vi "HFRR ADV v11.vi"() -> ()   [LabVIEW 2025] (continued)
            n1532 = local read "AIR TEMP INTERCEPT:"() -> (w2037:dbl)
            n1533 = case shown="\"0\", Default" "Calibrating" {
              tunnel: w2028 -> [w2082 _]
              tunnel: [w2082 w2083] -> w2027
              tunnel: w2026 -> [_ w2083]
              frame "0", Default {
              }
              frame "1" {
              }
            }
            n1534 = Multiply(x=w2016, y="ECR_Gain") -> (x*y=w2015:dbl)
            n1535 = Add(x=w2022, y=w2033) -> (x+y=w2038:dbl)
            n1536 = Multiply(x=w2056, y=79.77669138) -> (x*y=w2054:dbl)
            n1537 = Select(t=0.01 ("FF fil1"), s=w2053, f=0.1 ("FF fil1")) -> (s? t:f=w2049:dbl)
            n1538 = local read "ecr"() -> (w2010:dbl)
            n1539 = Multiply(x=w2021, y=w2041) -> (x*y=w2023:dbl)
            n1540 = Multiply(x=w2063, y=w2054) -> (x*y=w2060:dbl[])
            n1541 = Multiply(x=w2015, y=0.2) -> (x*y=w2008:dbl)
            n1542 = Multiply(x=0.8, y=w2010) -> (x*y=w2009:dbl)
            n1543 = call <vilib>:"Mean PtByPt.vi"("x"=w2038, "sample length"=10) -> ("mean"=w1999:dbl)  [unwired: 2 in, 1 out]
            "TEMP 2" <- w1999
            "TEMP 3" <- w1999
            n1544 = local read "AIR TEMP"() -> (w2046:dbl)
            n1545 = Add(x=w2023, y=w2037) -> (x+y=w2039:dbl)
            n1546 = call-poly <vilib>:"Mean.vi"("X"=w2060) -> ("mean"=w2061:dbl)  [unwired: 1 out]
            n1547 = Add(x=w2008, y=w2009) -> (x+y=w2007:dbl)
            n1548 = Subtract(x=1.0 ("y"), y=w2049) -> (x-y=w2047:dbl)
            n1549 = local write "TEMP"(w1999) -> ()
            n1550 = Multiply(x=w2047, y=w2046) -> (x*y=w2045:dbl)
            n1551 = Multiply(x=w2039, y=w2049) -> (x*y=w2050:dbl)
            n1552 = Not A Number/Path/Refnum?(number/path/refnum=w2007) -> (NaN/Path/Refnum?=w2017:bool)
            n1553 = Subtract(x=w2060, y=w2061) -> (x-y=w2032:dbl[])
            n1554 = local read "FRICVALZ"() -> (w2070:dbl)
            n1555 = case shown="True" "Camera Button" {
              tunnel: w2027 -> [_ w2089]
              tunnel: "Standard Temp. ( °c )" -> [_ w2088]
              frame False {
              }
              frame True {
                n1556 = Build Array(w2088, w2089) -> (w2087:dbl[])
                n1557 = local write "Camera Button"(FALSE ("Boolean 4")) -> ()
                n1558 = local read "Captured Values"() -> (w2086:dbl[][])
                n1559 = Build Array (concatenate)(w2086, w2087) -> (w2084:dbl[][])
                n1560 = local write "Captured Values"(w2084) -> ()
              }
            }
            n1561 = Compound Arithmetic op=OR("FRICVALZ 4", "FRICVALZ 3", "FRICVALZ 2") -> (w2001:bool)
            n1562 = Add(x=w2050, y=w2045) -> (x+y=w2043:dbl)
            n1563 = Absolute Value(x=w2032) -> (abs(x)=w2065:dbl[])
            n1564 = call-poly <vilib>:"RMS.vi"("X"=w2032) -> ("rms value"=w2031:dbl)  [unwired: 1 out]
            n1565 = Select(t=0.0, s=w2017, f=w2007) -> (s? t:f=w2014:dbl)
            n1566 = call-poly <vilib>:"Mean.vi"("X"=w2065) -> ()  [unwired: 2 out]
            n1567 = local read "FF 2"() -> (w2072:dbl)
            n1568 = case shown="True" w2001 {
              tunnel: w2031 -> [_ w2094]
              frame False {
              }
              frame True {
                w2093 = FALSE ("FRICVALZ")
                n1569 = local write "FRICVALZ 3"(w2093) -> ()
                n1570 = local write "FRICVALZ 2"(w2093) -> ()
                n1571 = local write "FRICVALZ 4"(w2093) -> ()
                "FRICVALZ" <- w2094
              }
            }
            n1572 = Subtract(x=w2031, y=w2070) -> (x-y=w2064:dbl)
            n1573 = Not A Number/Path/Refnum?(number/path/refnum=w2043) -> (NaN/Path/Refnum?=w2044:bool)
            n1574 = In Range and Coerce(upper limit=100.0, x=w2014, lower limit=0.0) -> ()  [unwired: 2 out]
            n1575 = Select(t=0.0, s=w2044, f=w2043) -> (s? t:f=w2004:dbl)
            "AIR TEMP" <- w2004
            n1576 = Multiply(x=w2064, y=0.1 ("FF fil1")) -> (x*y=w2076:dbl)
            n1577 = Multiply(x=0.9 ("FF fil2"), y=w2072) -> (x*y=w2075:dbl)
            n1578 = disable-structure shown="Disabled" {
              frame Disabled {
                n1579 = local read "NORMAL LOAD"() -> ()  [unwired: 1 out]
              }
              frame Enabled {
              }
            }
            n1580 = call "Elapsed Time11"("Time Target (s)"=1.0) -> ("Time has Elapsed"=w2006:bool)  [unwired: 11 in, 7 out]
            n1581 = Add(x=w2076, y=w2075) -> (x+y=w1994:dbl)
            "FF 2" <- w1994
            "FF 4" <- w1994
            n1582 = case shown="True" w2006 {
              tunnel: w2004 -> [_ w2078]
              frame False {
              }
              frame True {
                "AirT" <- w2078
              }
            }
            n1583 = local read "TEMP"() -> (w2069:dbl)
            n1584 = local write "FF 3"(w1994) -> ()
            n1585 = Not A Number/Path/Refnum?(number/path/refnum=w1994) -> (NaN/Path/Refnum?=w2067:bool)
            n1586 = Divide(x=w1994, y=1.96) -> (x/y=w2034:dbl)
            n1587 = Not A Number/Path/Refnum?(number/path/refnum=w2069) -> (NaN/Path/Refnum?=w2068:bool)
            n1588 = Compound Arithmetic op=OR(w2068, w2067) -> (w2066:bool)
            n1589 = Not A Number/Path/Refnum?(number/path/refnum=w2034) -> (NaN/Path/Refnum?=w2035:bool)
            n1590 = case shown="True" w2066 {
              frame False {
              }
              frame True {
                n1591 = local write "TEMP"(0.0 ("TEMP")) -> ()
                n1592 = local write "FF 2"(0.0 ("FF 2")) -> ()
                n1593 = local write "reinit"(TRUE ("reinit")) -> ()
              }
            }
            n1594 = Select(t=0.0, s=w2035, f=w2034) -> (s? t:f=w1995:dbl)
            "COF 2" <- w1995
            n1595 = local write "COF 3"(w1995) -> ()
          }
          frame #4 {
            n1596 = flat-sequence {
              frame #0 {
                n1597 = Wait (ms)(milliseconds to wait=u32 100) -> ()  [unwired: 1 out]
              }
              frame #1 {
                n1598 = local write "Lift"(FALSE ("Lift")) -> ()
              }
            }
            n1599 = case shown="True" "Calculate Button" {
              frame False {
              }
              frame True {
                n1600 = local write "Calculate Button"(FALSE ("Boolean 6")) -> ()
                n1601 = local read "Captured Values"() -> (w2105:dbl[][])
                n1602 = Index Array(array=w2105, index (col) #1=0 ("disabled index (col)"), index (col) #2=1 ("index (col)")) -> (element #1=w2103:dbl[], element #2=w2101:dbl[])  [unwired: 2 in]
                n1603 = call <vilib>:"Linear Fit.vi"("Y"=w2103, "X"=w2101) -> ("Best Linear Fit"=→"Best Fit":dbl[], "slope"=w2097:dbl, "intercept"=w2096:dbl)  [unwired: 9 in, 2 out]
                "Slope" <- w2097
                "Intercept" <- w2096
                n1604 = local read "Calibrating"() -> (w2098:string)
                n1605 = case shown="\"1\"" w2098 {
                  tunnel: w2097 -> [w2107 w2109]
                  tunnel: w2096 -> [w2106 w2108]
                  frame "0", Default {
                    n1606 = local write "TEMPERATURE :"(w2107) -> ()
                    n1607 = local write "TEMP INTERCEPT:"(w2106) -> ()
                  }
                  frame "1" {
                    n1608 = local write "AIR TEMPERATURE :"(w2109) -> ()
                    n1609 = local write "AIR TEMP INTERCEPT:"(w2108) -> ()
                  }
                }
              }
            }
          }
        }
      }
    }
    n1610 = Wait (ms)(milliseconds to wait=u32 50) -> ()  [unwired: 1 out]
    n1611 = local read "Quit"() -> (w1899:bool)
    "Rate" <- 2500.0 ("No of Samples")
    "Humid Last buf" <- dbl[] [0.0, 0.0, 0.0, 0.0] ("Humid Last buf")
  }
  n1612 = while {
    tunnel: w60 -> [_]
    tunnel: [w2139] -> _
    tunnel: [w2114] -> w57
    i -> [w2139]
    stop <- w2114 stop-if-true
    # "C:\\LAB-IQ-NXT\\Scar View.exe"
    n1613 = local read "OK Button 16"() -> (w2128:bool)
    n1614 = local read "Re-Initialise"() -> (w2124:bool)
    n1615 = local read "Main Tab"() -> (w2120:T2)
    n1616 = local read "service 3"() -> (w2121:bool)
    n1617 = local read "OPEN 6"() -> (w2123:bool)
    n1618 = local read "EDIT 2"() -> (w2126:bool)
    n1619 = flat-sequence {
      frame #0 {
        n1620 = local read "SAVE 2"() -> (w2742:bool)
        n1621 = stacked-sequence {
          frame #0 {
            n1622 = local read "EDIT"() -> (w2796:bool)
            n1623 = case shown="True" w2796 {
              tunnel: [u8 2 ("Disabled") u8 0 ("Disabled")] -> _
              frame False {
                w2798 = FALSE
                n1624 = local write "Password"("") -> ()
                n1625 = property on="SrvM CP" class="Bool (strict)"("Visible"=w2798) -> ()  [unwired: 2 in, 2 out]
                n1626 = property on="message" class="Str"("Visible"=w2798) -> ()  [unwired: 2 in, 2 out]
                n1627 = local write "x = y?"(w2798) -> ()
                n1628 = property on="Password" class="Str"("Visible"=w2798) -> ()  [unwired: 2 in, 2 out]
                n1629 = property on="ENTER THE NEW PASSWORD" class="Str"("Visible"=w2798) -> ()  [unwired: 2 in, 2 out]
                n1630 = property on="ENTER CURRENT PASSWORD" class="Str"("Visible"=w2798) -> ()  [unwired: 2 in, 2 out]
                n1631 = local write "SrvM CP"(w2798) -> ()
              }
              frame True {
                w2801 = TRUE
                n1632 = property on="SrvM CP" class="Bool (strict)"("Visible"=w2801) -> ()  [unwired: 2 in, 2 out]
                n1633 = property on="Password" class="Str"("Visible"=w2801) -> ()  [unwired: 2 in, 2 out]
              }
            }
            "dipl pwd" <- "@143$\n" ("dipl pwd")
          }
          frame #1 {
            # "Gain password"
            n1634 = String To Byte Array(string="ENTER CURRENT PASSWORD") -> (unsigned byte array=w2806:u8[])
            n1635 = Search 1D Array(1D array=w2806, element=u8 10) -> (index of element=w2809:i32)  [unwired: 1 in]
            n1636 = Index Array(array=w2806, index=w2809) -> (element=w2805:u8)
            n1637 = Equal?(x=w2805, y=10) -> (x = y?=w2803:bool)
            n1638 = case shown="True" w2803 {
              frame False {
                n1639 = property on="ENTER THE NEW PASSWORD" class="Str"("Visible"=FALSE) -> ()  [unwired: 2 in, 2 out]
              }
              frame True {
                # "password"
                # "change password logic"
                n1640 = local read "ENTER CURRENT PASSWORD"() -> (w2822:string)
                n1641 = local read "dipl pwd"() -> (w2816:string)
                n1642 = String To Byte Array(string=w2822) -> (unsigned byte array=w2824:u8[])
                n1643 = String To Byte Array(string=w2816) -> (unsigned byte array=w2817:u8[])
                n1644 = Array Size(array=w2824) -> (size(s)=w2821:i32)
                n1645 = Array Size(array=w2817) -> (size(s)=w2819:i32)
                n1646 = for {
                  N: w2821 -> [_]
                  tunnel: w2824 -> [w2848]
                  tunnel: [w2846] -> w2825 mode=indexing
                  tunnel: w2821 -> [w2840]
                  i -> [w2841]
                  n1647 = Decrement(x=w2840) -> (x-1=w2838:i32)
                  n1648 = Equal?(x=w2841, y=w2838) -> (x = y?=w2839:bool)
                  n1649 = Index Array(array=w2848, index=w2841) -> (element=w2842:u8)
                  n1650 = Number To Decimal String(number=w2842) -> (decimal integer string=w2847:string)  [unwired: 1 in]
                  n1651 = Select(t="", s=w2839, f="\r") -> (s? t:f=w2844:string)
                  n1652 = Concatenate Strings(w2847, w2844) -> (w2846:string)
                }
                n1653 = for {
                  N: w2819 -> [_]
                  tunnel: w2817 -> [w2836]
                  tunnel: [w2834] -> w2818 mode=indexing
                  tunnel: w2819 -> [w2831]
                  i -> [w2832]
                  n1654 = Decrement(x=w2831) -> (x-1=w2830:i32)
                  n1655 = Equal?(x=w2832, y=w2830) -> (x = y?=w2829:bool)
                  n1656 = Index Array(array=w2836, index=w2832) -> (element=w2835:u8)
                  n1657 = Number To Decimal String(number=w2835) -> (decimal integer string=w2833:string)  [unwired: 1 in]
                  n1658 = Select(t="", s=w2829, f="\r") -> (s? t:f=w2826:string)
                  n1659 = Concatenate Strings(w2833, w2826) -> (w2834:string)
                }
                n1660 = local read "string"() -> (w2823:string)
                n1661 = Concatenate Strings(w2818) -> (w2812:string)
                n1662 = Concatenate Strings(w2823) -> (w2820:string)
                n1663 = Concatenate Strings(w2825) -> (w2813:string)
                n1664 = Equal?(x=w2813, y=w2820) -> (x = y?=w2815:bool)
                n1665 = Equal?(x=w2813, y=w2812) -> (x = y?=w2811:bool)
                n1666 = Or(x=w2815, y=w2811) -> (x .or. y?=w2814:bool)
                n1667 = case shown="True" w2814 {
                  frame False {
                  }
                  frame True {
                    n1668 = property on="ENTER THE NEW PASSWORD" class="Str"("Visible"=TRUE) -> ()  [unwired: 2 in, 2 out]
                  }
                }
              }
            }
          }
          frame #2 {
            n1669 = String To Byte Array(string="ENTER THE NEW PASSWORD") -> (unsigned byte array=w2851:u8[])
            n1670 = Search 1D Array(1D array=w2851, element=u8 10) -> (index of element=w2855:i32)  [unwired: 1 in]
            n1671 = Index Array(array=w2851, index=w2855) -> (element=w2853:u8)
            n1672 = Equal?(x=w2853, y=10) -> (x = y?=w2850:bool)
            n1673 = case shown="False" w2850 {
              frame False {
              }
              frame True {
                n1674 = local write "EDIT"(FALSE) -> ()
                n1675 = local write "SrvM CP"(FALSE) -> ()
                n1676 = local read "ENTER THE NEW PASSWORD"() -> (w2858:string)
                n1677 = String To Byte Array(string=w2858) -> (unsigned byte array=w2863:u8[])
                n1678 = Array Size(array=w2863) -> (size(s)=w2860:i32)
                n1679 = for {
                  N: w2860 -> [_]
                  tunnel: w2863 -> [w2876]
                  tunnel: [w2873] -> w2865 mode=indexing
                  tunnel: w2860 -> [w2868]
                  i -> [w2866]
                  n1680 = Decrement(x=w2868) -> (x-1=w2869:i32)
                  n1681 = Equal?(x=w2866, y=w2869) -> (x = y?=w2870:bool)
                  n1682 = Index Array(array=w2876, index=w2866) -> (element=w2875:u8)
                  n1683 = Number To Decimal String(number=w2875) -> (decimal integer string=w2874:string)  [unwired: 1 in]
                  n1684 = Select(t="", s=w2870, f="\r") -> (s? t:f=w2867:string)
                  n1685 = Concatenate Strings(w2874, w2867) -> (w2873:string)
                }
                n1686 = local read "file path"() -> (w2857:path)
                n1687 = Concatenate Strings(w2865) -> (w2859:string)
                n1688 = Delete(path (use dialog)=w2857) -> (deleted path=w2861:path)  [unwired: 4 in, 2 out]
                n1689 = call <vilib>:"Write Characters To File.vi"("append to file? (new file:F)"=FALSE, "character string"=w2859, "file path (dialog if empty)"=w2861) -> ()  [unwired: 2 in, 1 out]
              }
            }
          }
          frame #3 {
            n1690 = case shown="True" "SrvM CP" {
              frame False {
                w2879 = ""
                n1691 = local write "ENTER CURRENT PASSWORD"(w2879) -> ()
                n1692 = local write "ENTER THE NEW PASSWORD"(w2879) -> ()
                n1693 = property on="ENTER CURRENT PASSWORD" class="Str"("Visible"=FALSE) -> ()  [unwired: 2 in, 2 out]
              }
              frame True {
                n1694 = property on="ENTER THE NEW PASSWORD" class="Str"() -> ("Visible"=w2880:bool)  [unwired: 2 in, 2 out]
                n1695 = Not(x=w2880) -> (.not. x?=w2881:bool)
                n1696 = property on="ENTER CURRENT PASSWORD" class="Str"("Visible"=w2881) -> ()  [unwired: 2 in, 2 out]
              }
            }
          }
          frame #4 {
            n1697 = String To Byte Array(string="Password") -> (unsigned byte array=w2888:u8[])
            n1698 = Search 1D Array(1D array=w2888, element=u8 10) -> (index of element=w2886:i32)  [unwired: 1 in]
            n1699 = Index Array(array=w2888, index=w2886) -> (element=w2887:u8)
            n1700 = Equal?(x=w2887, y=10) -> (x = y?=w2883:bool)
            n1701 = case shown="True" w2883 {
              frame False {
              }
              frame True {
                # "password"
                # "password"
                n1702 = local read "Password"() -> (w2901:string)
                n1703 = String To Byte Array(string=w2901) -> (unsigned byte array=w2904:u8[])
                n1704 = String To Byte Array(string="@143$\n") -> (unsigned byte array=w2890:u8[])
                n1705 = Array Size(array=w2904) -> (size(s)=w2899:i32)
                n1706 = Array Size(array=w2890) -> (size(s)=w2895:i32)
                n1707 = for {
                  N: w2899 -> [_]
                  tunnel: w2904 -> [w2938]
                  tunnel: [w2936] -> w2905 mode=indexing
                  tunnel: w2899 -> [w2933]
                  i -> [w2934]
                  n1708 = Decrement(x=w2933) -> (x-1=w2932:i32)
                  n1709 = Index Array(array=w2938, index=w2934) -> (element=w2937:u8)
                  n1710 = Equal?(x=w2934, y=w2932) -> (x = y?=w2931:bool)
                  n1711 = Number To Decimal String(number=w2937) -> (decimal integer string=w2935:string)  [unwired: 1 in]
                  n1712 = Select(t="", s=w2931, f="\r") -> (s? t:f=w2928:string)
                  n1713 = Concatenate Strings(w2935, w2928) -> (w2936:string)
                }
                n1714 = for {
                  N: w2895 -> [_]
                  tunnel: w2890 -> [w2949]
                  tunnel: [w2947] -> w2893 mode=indexing
                  tunnel: w2895 -> [w2944]
                  i -> [w2945]
                  n1715 = Decrement(x=w2944) -> (x-1=w2943:i32)
                  n1716 = Index Array(array=w2949, index=w2945) -> (element=w2948:u8)
                  n1717 = Equal?(x=w2945, y=w2943) -> (x = y?=w2942:bool)
                  n1718 = Number To Decimal String(number=w2948) -> (decimal integer string=w2946:string)  [unwired: 1 in]
                  n1719 = Select(t="", s=w2942, f="\r") -> (s? t:f=w2939:string)
                  n1720 = Concatenate Strings(w2946, w2939) -> (w2947:string)
                }
                n1721 = local read "file path"() -> (w2889:path)
                n1722 = call <vilib>:"Read Characters From File.vi"("file path (dialog if empty)"=w2889) -> ("character string"=w2903:string)  [unwired: 5 in, 3 out]
                "string" <- w2903
                n1723 = flat-sequence {
                  tunnel: [w2906] -> w2900
                  frame #0 {
                    w2906 = ""
                    n1724 = local write "Password"(w2906) -> ()
                  }
                }
                n1725 = Concatenate Strings(w2893) -> (w2894:string)
                n1726 = Concatenate Strings(w2903) -> (w2902:string)
                n1727 = Concatenate Strings(w2905) -> (w2897:string)
                n1728 = Equal?(x=w2897, y=w2902) -> (x = y?=w2892:bool)
                n1729 = Equal?(x=w2897, y=w2894) -> (x = y?=w2898:bool)
                n1730 = Or(x=w2892, y=w2898) -> (x .or. y?=w2891:bool)
                "x = y?" <- w2891
                n1731 = case shown="True" w2891 {
                  selector: w2891 -> [w2908 _]
                  tunnel: w2900 -> [_ _]
                  frame False {
                    n1732 = And(x=w2908, y=TRUE ("Visible")) -> (x .and. y?=w2909:bool)
                    n1733 = property on="message" class="Str"("Visible"=w2909) -> ()  [unwired: 2 in, 2 out]
                  }
                  frame True {
                    n1734 = control-ref of="This VI"() -> (w2920:refnum<vi>)
                    n1735 = property class="VI"(reference=w2920) -> (reference out=w2911:refnum<vi>, error out=w2915:errorcluster, "Panel"=w2919:refnum<vi>)  [unwired: 1 in]
                    n1736 = property on="message" class="Str"("Visible"=FALSE) -> ()  [unwired: 2 in, 2 out]
                    n1737 = property class="Pnl"(reference=w2919, error in=w2915) -> (reference out=w2913:refnum<vi>, error out=w2916:errorcluster, "Panes[]"=w2918:refnum<vi>[])
                    n1738 = for {
                      tunnel: w2918 -> [w2927] mode=indexing
                      tunnel: T18."Always On" ("Horizontal Scrollbar Visibility") -> [w2926]
                      tunnel: w2916 -> [w2923]
                      tunnel: [w2922] -> w2914
                      n1739 = property class="Pane"(reference=w2927, error in=w2923, "HorizScrollbarVisibility"=w2926) -> (reference out=w2924:refnum<vi>, error out=w2925:errorcluster)
                      n1740 = Close Reference(reference=w2924, error in (no error)=w2925) -> (error out=w2922:errorcluster)
                    }
                    n1741 = Close Reference(reference=w2913, error in (no error)=w2914) -> (error out=w2912:errorcluster)
                    n1742 = Close Reference(reference=w2911, error in (no error)=w2912) -> (error out=→"error out 6":errorcluster)
                  }
                }
              }
            }
          }
        }
        n1743 = local read "x = y?"() -> (w2748:bool)
        n1744 = local read "HUMIDITY: 2"() -> (w2750:dbl)
        n1745 = local read "HUMIDITY:"() -> (w2749:dbl)
        n1746 = property on="Port 2 Error" class="Clust (strict)"("Visible"="EDIT") -> ()  [unwired: 2 in, 2 out]
        n1747 = property on="Port 1 Error" class="Clust (strict)"("Visible"="EDIT") -> ()  [unwired: 2 in, 2 out]
        n1748 = case shown="True" "SrvM CP 2" {
          frame False {
          }
          frame True {
            n1749 = local write "SrvM CP 2"(FALSE ("SrvM CP 2")) -> ()
            n1750 = local read "HUMIDITY: 2"() -> (w2789:dbl)
            n1751 = local read "TEMP INTERCEPT: 2"() -> (w2788:dbl)
            n1752 = local read "DISPLACEMENT : 4"() -> (w2792:dbl)
            n1753 = local read "TEMPERATURE : 2"() -> (w2791:dbl)
            n1754 = local read "STROKE GAIN : 2"() -> (w2793:dbl)
            n1755 = local read "FRIC. FORCE : 2"() -> (w2794:dbl)
            n1756 = local read "AIR TEMP INTERCEPT: 2"() -> (w2787:dbl)
            n1757 = local read "AIR TEMPERATURE : 2"() -> (w2790:dbl)
            n1758 = local write "HUMIDITY:"(w2789) -> ()
            n1759 = local write "AIR TEMP INTERCEPT:"(w2788) -> ()
            n1760 = local write "TEMPERATURE :"(w2791) -> ()
            n1761 = local write "FRIC. FORCE :"(w2794) -> ()
            n1762 = local write "STROKE GAIN :"(w2793) -> ()
            n1763 = local write "DISPLACEMENT :"(w2792) -> ()
            n1764 = local write "AIR TEMPERATURE :"(w2790) -> ()
            n1765 = local write "TEMP INTERCEPT:"(w2787) -> ()
          }
        }
        n1766 = Or(x="SAVE", y=w2742) -> (x .or. y?=w2743:bool)
        n1767 = And(x="EDIT", y=w2748) -> (x .and. y?=w2746:bool)
        n1768 = local read "DISPLACEMENT : 4"() -> (w2759:dbl)
        n1769 = local read "TEMPERATURE : 2"() -> (w2757:dbl)
        n1770 = local read "STROKE GAIN : 2"() -> (w2763:dbl)
        n1771 = local read "DISPLACEMENT :"() -> (w2758:dbl)
        n1772 = local read "FRIC. FORCE : 2"() -> (w2766:dbl)
        n1773 = local read "TEMPERATURE :"() -> (w2755:dbl)
        n1774 = local read "STROKE GAIN :"() -> (w2762:dbl)
        n1775 = local read "FRIC. FORCE :"() -> (w2765:dbl)
        n1776 = case shown="True" w2746 {
          tunnel: [u8 2 ("Disabled") u8 0 ("Disabled")] -> w2745
          tunnel: [w3136 TRUE ("Visible")] -> w2744
          frame False {
            w3136 = FALSE ("Visible")
            n1777 = local write "EDIT 2"(w3136) -> ()
          }
          frame True {
          }
        }
        n1778 = case shown="True" w2743 {
          frame False {
          }
          frame True {
            n1779 = stacked-sequence {
              seq-local: [w2966 _ _] -> [_ w3130 _]
              frame #0 {
                (unwired) i16 5 ("precision (6)")
                # "[CH1]    - FF\n[CH2]   - TEMPERATURE\n[CH3]    - Humidity\n[CH4]    - AIR TEMP\n[CH5]\\- Visa Uno\n[CH6] \\- Visa Due\n[CH7]  \\- file path\n[CH8]   - Displacement Gain\n[CHA]   - Stroke Gain\n[CHB]   - Stroke PID Gain\n[CHC]   -Language Selection\n[CHD]   -Power +\n[CHE]   -Power_\n[CHF]   -Heater\n[CHG]   -Humidity Wet\n[CHH]   -Humidity Dry\n[CHI]   -Integral Time"
                n1780 = local read "Stroke PID Gains"() -> (w3017:T9)
                n1781 = Unbundle By Name(w3017) -> ("Proportional Gain (Kc)"=w3016:dbl, "Integral Time (Ti, min)"=w2958:dbl)
                n1782 = Number To Fractional String(number=w2958, width (-)=i16 10 ("precision (6)"), precision (6)=i16 5) -> (F-format string=w2962:string)  [unwired: 1 in]
                n1783 = local read "Language Selection"() -> (w3014:enum16{"English", "Russian"})
                n1784 = local read "CH-HUMIDITY WET"() -> (w2972:u16)
                n1785 = local read "CH-HUMIDITY DRY"() -> (w2969:u16)
                n1786 = local read "STROKE GAIN :"() -> (w2950:dbl)
                n1787 = local read "CH-POWER +"() -> (w2981:u16)
                n1788 = local read "CH-POWER -"() -> (w2978:u16)
                n1789 = local read "CH-HEATER"() -> (w2975:u16)
                n1790 = local read "AIR TEMPERATURE :"() -> (w2953:dbl)
                n1791 = Concatenate Strings("[CHI]" ("string"), w2962, "-Integral Time " ("string"), "\r") -> (w2959:string)
                n1792 = local read "DISPLACEMENT :"() -> (w2951:dbl)
                n1793 = local read "TEMPERATURE :"() -> (w2954:dbl)
                n1794 = local read "FRIC. FORCE :"() -> (w2955:dbl)
                n1795 = local read "HUMIDITY:"() -> (w2952:dbl)
                n1796 = Path To String(path="File Path") -> (string=w3039:string)
                n1797 = Number To Fractional String(number=w2950, width (-)=i16 10 ("precision (6)"), precision (6)=i16 5) -> (F-format string=w3030:string)  [unwired: 1 in]
                n1798 = Number To Fractional String(number=w3016, width (-)=i16 10 ("precision (6)"), precision (6)=i16 5) -> (F-format string=w3018:string)  [unwired: 1 in]
                n1799 = Number To Fractional String(number=w3014, width (-)=i16 10 ("precision (6)"), precision (6)=i16 5) -> (F-format string=w3010:string)  [unwired: 1 in]
                n1800 = Number To Fractional String(number=w2981, width (-)=i16 10 ("precision (6)"), precision (6)=i16 5) -> (F-format string=w3004:string)  [unwired: 1 in]
                n1801 = Number To Fractional String(number=w2978, width (-)=i16 10 ("precision (6)"), precision (6)=i16 5) -> (F-format string=w3001:string)  [unwired: 1 in]
                n1802 = Number To Fractional String(number=w2975, width (-)=i16 10 ("precision (6)"), precision (6)=i16 5) -> (F-format string=w2996:string)  [unwired: 1 in]
                n1803 = Number To Fractional String(number=w2972, width (-)=i16 10 ("precision (6)"), precision (6)=i16 5) -> (F-format string=w2993:string)  [unwired: 1 in]
                n1804 = Number To Fractional String(number=w2969, width (-)=i16 10 ("precision (6)"), precision (6)=i16 5) -> (F-format string=w2988:string)  [unwired: 1 in]
                n1805 = local read "Com Port 1"() -> (w2957:refnum<visa-resource-name>)
                n1806 = local read "Com Port 2"() -> (w2956:refnum<visa-resource-name>)
                n1807 = Concatenate Strings(w3039, "\\" ("string")) -> (w3038:string)
                n1808 = Number To Fractional String(number=w2955, width (-)=i16 10 ("precision (6)"), precision (6)=i16 5) -> (F-format string=w3071:string)  [unwired: 1 in]
                n1809 = Number To Fractional String(number=w2954, width (-)=i16 10 ("precision (6)"), precision (6)=i16 5) -> (F-format string=w3070:string)  [unwired: 1 in]
                n1810 = Number To Fractional String(number=w2952, width (-)=i16 10 ("precision (6)"), precision (6)=i16 5) -> (F-format string=w3064:string)  [unwired: 1 in]
                n1811 = Number To Fractional String(number=w2953, width (-)=i16 10 ("precision (6)"), precision (6)=i16 5) -> (F-format string=w3058:string)  [unwired: 1 in]
                n1812 = Number To Fractional String(number=w2951, width (-)=i16 10 ("precision (6)"), precision (6)=i16 5) -> (F-format string=w3031:string)  [unwired: 1 in]
                n1813 = Concatenate Strings("[CHA]" ("string"), w3030, "- Stroke Gain" ("string"), "\r") -> (w3024:string)
                n1814 = Concatenate Strings("[CHB]" ("string"), w3018, "- Stroke PID Gain" ("string"), "\r") -> (w3015:string)
                n1815 = Concatenate Strings("[CHC]" ("string"), w3010, "-Language Selection" ("string"), "\r") -> (w3007:string)
                n1816 = Concatenate Strings("[CHD]" ("string"), w3004, "-Power +" ("string"), "\r") -> (w2986:string)
                n1817 = Concatenate Strings("[CHG]" ("string"), w2993, "-Humidity Wet" ("string"), "\r") -> (w2983:string)
                n1818 = Concatenate Strings("[CHH]" ("string"), w2988, "-Humidity Dry" ("string"), "\r") -> (w2982:string)
                n1819 = Concatenate Strings("[CH1]" ("string"), w3071, " - FF" ("string"), "\r") -> (w3069:string)
                n1820 = Concatenate Strings("[CH2]" ("string"), w3070, " - TEMPERATURE" ("string"), "\r") -> (w3068:string)
                n1821 = Concatenate Strings("[CH3]" ("string"), w3064, " - Humidity" ("string"), "\r") -> (w3061:string)
                n1822 = Concatenate Strings("[CH4]" ("string"), w3058, " - AIR TEMP" ("string"), "\r") -> (w3054:string)
                n1823 = Concatenate Strings("[CH5]" ("string"), w2957, "- Visa Uno" ("string"), "\r") -> (w3047:string)
                n1824 = Concatenate Strings("[CH6]" ("string"), w2956, "- Visa Due" ("string"), "\r") -> (w3042:string)
                n1825 = Concatenate Strings("[CH7]" ("string"), w3038, "- file path" ("string"), "\r") -> (w3041:string)
                n1826 = Concatenate Strings("[CH8]" ("string"), w3031, "- Displacement Gain" ("string"), "\r") -> (w3034:string)
                n1827 = Concatenate Strings("[CHE]" ("string"), w3001, "-Power_" ("string"), "\r") -> (w2985:string)
                n1828 = Concatenate Strings("[CHF]" ("string"), w2996, "-Heater" ("string"), "\r") -> (w2984:string)
                n1829 = Concatenate Strings(w3069, w3068, w3061, w3054, w3047, w3042, w3041, w3034, w3024, w3015, w3007, w2986, w2985, w2984, w2983, w2982, w2959) -> (w2966:string)
                "gain" <- w2966
              }
              frame #1 {
                n1830 = local read "Camera Port :"() -> (w3083:string)
                n1831 = local read "TEMP INTERCEPT:"() -> (w3092:dbl)
                n1832 = local read "AIR TEMP INTERCEPT:"() -> (w3093:dbl)
                n1833 = local read "C3 :"() -> (w3091:refnum<visa-resource-name>)
                n1834 = local read "LvdtOff"() -> (w3095:dbl)
                n1835 = Number To Fractional String(number=w3092, width (-)=i16 10 ("precision (6)"), precision (6)=i16 5) -> (F-format string=w3118:string)  [unwired: 1 in]
                n1836 = local read "Com Port 3"() -> (w3102:refnum<visa-resource-name>)
                n1837 = Concatenate Strings("[CH8]" ("string"), w3083, "- Visa Camera" ("string"), "\r") -> (w3082:string)
                n1838 = Concatenate Strings("[CH7]" ("string"), w3091, "- Visa Humidity" ("string"), "\r") -> (w3087:string)
                n1839 = Number To Fractional String(number=w3093, width (-)=i16 10 ("precision (6)"), precision (6)=i16 5) -> (F-format string=w3125:string)  [unwired: 1 in]
                n1840 = Number To Fractional String(number=w3095, width (-)=i16 10 ("precision (6)"), precision (6)=i16 5) -> (F-format string=w3099:string)  [unwired: 1 in]
                n1841 = Concatenate Strings("[CHK]" ("string"), w3118, "-TEMP INTERCEPT" ("string"), "\r") -> (w3114:string)
                n1842 = Concatenate Strings("[SNO]" ("string"), "S.NO", "-" ("string"), "\r") -> (w3110:string)
                n1843 = Concatenate Strings("[CHI]" ("string"), w3099, "-LVDT Position Offset" ("string"), "\r") -> (w3094:string)
                n1844 = Concatenate Strings("[CHJ]" ("string"), w3125, "-AIR TEMP INTERCEPT" ("string"), "\r") -> (w3115:string)
                n1845 = Concatenate Strings("[CHL]" ("string"), w3102, "- Visa humid" ("string"), "\r") -> (w3105:string)
                n1846 = String To Path(string="C:\\LAB-IQ\\calibrate WO 2465.dcf") -> (path=w3103:path)
                n1847 = Concatenate Strings(w3130, w3115, w3114, w3110, w3105, w3094, w3087, w3082) -> (w3129:string)
                n1848 = call <vilib>:"Write Characters To File.vi"("append to file? (new file:F)"=FALSE, "character string"=w3129, "file path (dialog if empty)"=w3103) -> ()  [unwired: 2 in, 1 out]
              }
              frame #2 {
                n1849 = local write "Lan flag"(0.0 ("Lan flag")) -> ()
                n1850 = local write "conststatus"(0.0 ("rpm value : 2")) -> ()
                n1851 = local write "SAVE"(FALSE ("OK Button 14")) -> ()
                n1852 = local write "Re-Initialise"(TRUE ("Re-Initialise")) -> ()
                n1853 = local write "SAVE 2"(FALSE ("SAVE 2")) -> ()
              }
            }
          }
        }
        n1854 = Subtract(x=w2750, y=w2749) -> (x-y=w2751:dbl)
        n1855 = local read "AIR TEMPERATURE : 2"() -> (w2754:dbl)
        n1856 = local read "AIR TEMPERATURE :"() -> (w2753:dbl)
        n1857 = Divide(x=w2751, y=w2749) -> (x/y=w2773:dbl)
        n1858 = Subtract(x=w2766, y=w2765) -> (x-y=w2764:dbl)
        n1859 = Subtract(x=w2757, y=w2755) -> (x-y=w2756:dbl)
        n1860 = Subtract(x=w2763, y=w2762) -> (x-y=w2761:dbl)
        n1861 = Subtract(x=w2759, y=w2758) -> (x-y=w2760:dbl)
        n1862 = Subtract(x=w2754, y=w2753) -> (x-y=w2752:dbl)
        n1863 = Divide(x=w2764, y=w2765) -> (x/y=w2784:dbl)
        n1864 = Divide(x=w2756, y=w2755) -> (x/y=w2777:dbl)
        n1865 = Divide(x=w2761, y=w2762) -> (x/y=w2781:dbl)
        n1866 = Divide(x=w2760, y=w2758) -> (x/y=w2780:dbl)
        n1867 = Multiply(x=w2773, y=100.0) -> (x*y=→"HUMIDITY  Calibration Error":dbl)
        n1868 = Divide(x=w2752, y=w2753) -> (x/y=w2776:dbl)
        n1869 = Multiply(x=w2784, y=100.0) -> (x*y=→"FRIC. FORCE Calibration Error":dbl)
        n1870 = Multiply(x=w2777, y=100.0) -> (x*y=→"TEMPERATURE  Calibration Error":dbl)
        n1871 = Multiply(x=w2781, y=100.0) -> (x*y=→"STROKE Calibration Error":dbl)
        n1872 = Multiply(x=w2780, y=100.0) -> (x*y=→"DISPLACEMENT  Calibration Error":dbl)
        n1873 = property on="EDIT 2" class="Bool (strict)"("Visible"=w2744) -> ()  [unwired: 2 in, 2 out]
        n1874 = property on="SAVE" class="Bool (strict)"("Visible"=w2744) -> ()  [unwired: 2 in, 2 out]
        n1875 = property on="SrvM CP" class="Bool (strict)"("Disabled"=w2745) -> ()  [unwired: 2 in, 2 out]
        n1876 = property on="visa due" class="CmbBox"("Disabled"=w2745) -> ()  [unwired: 2 in, 2 out]
        n1877 = property on="LvdtOff" class="DigNum (strict)"("Disabled"=w2745) -> ()  [unwired: 2 in, 2 out]
        n1878 = property on="File Path" class="Path"("Disabled"=w2745) -> ()  [unwired: 2 in, 2 out]
        n1879 = Multiply(x=w2776, y=100.0) -> (x*y=→"AIR TEMPERATURE  Calibration Error":dbl)
        n1880 = property on="Tab Control" class="TabCtl (strict)"("Visible"=w2744) -> ()  [unwired: 2 in, 2 out]
        n1881 = property on="Language Selection" class="Enum (strict)"("Visible"=w2744) -> ()  [unwired: 2 in, 2 out]
        n1882 = property on="Tab Control 7" class="TabCtl (strict)"("Disabled"=w2745) -> ()  [unwired: 2 in, 2 out]
        n1883 = property on="AIR TEMP INTERCEPT:" class="DigNum (strict)"("Disabled"=w2745) -> ()  [unwired: 2 in, 2 out]
        n1884 = property on="CH-POWER -" class="DigNum (strict)"("Disabled"=w2745) -> ()  [unwired: 2 in, 2 out]
        n1885 = property on="CH-POWER +" class="DigNum (strict)"("Disabled"=w2745) -> ()  [unwired: 2 in, 2 out]
        n1886 = property on="AIR TEMPERATURE :" class="DigNum (strict)"("Disabled"=w2745) -> ()  [unwired: 2 in, 2 out]
        n1887 = property on="STROKE GAIN :" class="DigNum (strict)"("Disabled"=w2745) -> ()  [unwired: 2 in, 2 out]
        n1888 = property on="SPEED OUT:" class="DigNum (strict)"("Disabled"=w2745) -> ()  [unwired: 2 in, 2 out]
        n1889 = property on="CH-HUMIDITY DRY" class="DigNum (strict)"("Disabled"=w2745) -> ()  [unwired: 2 in, 2 out]
        n1890 = property on="HUMIDITY:" class="DigNum (strict)"("Disabled"=w2745) -> ()  [unwired: 2 in, 2 out]
        n1891 = property on="CH-HUMIDITY WET" class="DigNum (strict)"("Disabled"=w2745) -> ()  [unwired: 2 in, 2 out]
        n1892 = property on="Stroke PID Gains" class="Clust (strict)"("Disabled"=w2745) -> ()  [unwired: 2 in, 2 out]
        n1893 = property on="TEMPERATURE :" class="DigNum (strict)"("Disabled"=w2745) -> ()  [unwired: 2 in, 2 out]
        n1894 = property on="DISPLACEMENT :" class="DigNum (strict)"("Disabled"=w2745) -> ()  [unwired: 2 in, 2 out]
        n1895 = property on="CH-HEATER" class="DigNum (strict)"("Disabled"=w2745) -> ()  [unwired: 2 in, 2 out]
        n1896 = property on="TEMP INTERCEPT:" class="DigNum (strict)"("Disabled"=w2745) -> ()  [unwired: 2 in, 2 out]
        n1897 = property on="FRIC. FORCE :" class="DigNum (strict)"("Disabled"=w2745) -> ()  [unwired: 2 in, 2 out]
      }
    }
    n1898 = local read "RUN"() -> (w2138:bool)
    n1899 = local read "RUN"() -> (w2136:bool)
    n1900 = disable-structure shown="Disabled" {
      disable-tunnel: [w2153 _] -> w2118
      disable-tunnel: [w2152 _] -> w2116
      frame Disabled {
        n1901 = local read "Temperature before test"() -> (w2146:dbl)
        n1902 = local read "Temperature after test"() -> (w2159:dbl)
        n1903 = case shown="True" "Save Results" {
          frame False {
          }
          frame True {
            w2175 = "\r"
            n1904 = local write "Save Results"(FALSE ("OK Button 5")) -> ()
            n1905 = local read "Temperature before test"() -> (w2213:dbl)
            n1906 = local read "Temperature after test"() -> (w2215:dbl)
            n1907 = local read "Humidity before test"() -> (w2212:dbl)
            n1908 = local read "Humidity after test"() -> (w2214:dbl)
            n1909 = local read "WS1.4"() -> (w2219:dbl)
            n1910 = local read "AVP"() -> (w2217:dbl)
            n1911 = Number To Fractional String(number=w2219, width (-)=i16 6, precision (6)=i16 1) -> (F-format string=w2179:string)  [unwired: 1 in]
            n1912 = local read "MWSD"() -> (w2216:dbl)
            n1913 = local read "String"() -> (w2208:string)
            n1914 = local read "FILE"() -> (w2211:string)
            n1915 = local read "HCF"() -> (w2218:dbl)
            n1916 = Number To Fractional String(number=w2212, width (-)=i16 6, precision (6)=i16 1) -> (F-format string=w2204:string)  [unwired: 1 in]
            n1917 = Number To Fractional String(number=w2213, width (-)=i16 6, precision (6)=i16 1) -> (F-format string=w2201:string)  [unwired: 1 in]
            n1918 = Number To Fractional String(number=w2214, width (-)=i16 6, precision (6)=i16 1) -> (F-format string=w2197:string)  [unwired: 1 in]
            n1919 = Number To Fractional String(number=w2215, width (-)=i16 6, precision (6)=i16 1) -> (F-format string=w2193:string)  [unwired: 1 in]
            n1920 = Number To Fractional String(number=w2217, width (-)=i16 6, precision (6)=i16 3) -> (F-format string=w2186:string)  [unwired: 1 in]
            n1921 = Concatenate Strings(w2208, w2211) -> (w2230:string)
            n1922 = Number To Fractional String(number=w2216, width (-)=i16 6, precision (6)=i16 1) -> (F-format string=w2190:string)  [unwired: 1 in]
            n1923 = Number To Fractional String(number=w2218, width (-)=i16 6, precision (6)=i16 2) -> (F-format string=w2184:string)  [unwired: 1 in]
            n1924 = Concatenate Strings("(" ("string"), w2179, ")Microns" ("string")) -> (w2178:string)
            n1925 = local read "REMARKS"() -> (w2210:string)
            "REMARKS 2" <- w2210
            n1926 = Concatenate Strings("(" ("string"), w2204, " ) % RH," ("string")) -> (w2205:string)
            n1927 = Concatenate Strings(w2184, ")" ("string")) -> (w2182:string)
            n1928 = Concatenate Strings("(" ("string"), w2201, ")  Deg C ," ("string")) -> (w2200:string)
            n1929 = Concatenate Strings("(" ("string"), w2197, " ) % RH," ("string")) -> (w2196:string)
            n1930 = Concatenate Strings("(" ("string"), w2193, ")  Deg C ," ("string")) -> (w2192:string)
            n1931 = Concatenate Strings("(" ("string"), w2190, ")  Microns," ("string")) -> (w2189:string)
            n1932 = Concatenate Strings("(" ("string"), w2186, ")  kPa," ("string")) -> (w2176:string)
            n1933 = Concatenate Strings(w2230, ".dwm" ("Substring")) -> (w2228:string)
            n1934 = String To Path(string=w2228) -> (path=w2227:path)
            n1935 = Concatenate Strings(w2210, w2175, " Humidity before test= " ("Substring"), w2205, w2175, " Temperature before test = " ("Substring"), w2200, w2175, " Humidity after test= " ("Substring"), w2196, w2175, "Temperature after test = " ("Substring"), w2192, w2175, "MSD = " ("Substring"), w2189, w2175, "  AVP = " ("Substring"), w2176, w2175, "  HCF                     =( " ("Substring"), w2182, w2175, " WS1.4                  = " ("Substring"), w2178, w2175) -> (w2174:string)
            "data" <- w2174
            n1936 = call <vilib>:"Write Characters To File.vi"("append to file? (new file:F)"=FALSE, "character string"=w2174, "file path (dialog if empty)"=w2227) -> ()  [unwired: 2 in, 1 out]
            n1937 = Match Pattern(string=w2174, regular expression="!") -> (after substring=→"export":string)  [unwired: 1 in, 3 out]
          }
        }
        n1938 = Add(x=231.864, y=w2146) -> (x+y=w2143:dbl)
        n1939 = Add(x=231.864, y=w2159) -> (x+y=w2156:dbl)
        n1940 = Divide(x=1705.984, y=w2143) -> (x/y=w2144:dbl)
        n1941 = Divide(x=1705.984, y=w2156) -> (x/y=w2157:dbl)
        n1942 = local read "Humidity before test"() -> (w2148:dbl)
        n1943 = local read "Humidity after test"() -> (w2161:dbl)
        n1944 = Subtract(x=8.017352 ("y"), y=w2144) -> (x-y=w2170:dbl)
        n1945 = Subtract(x=8.017352 ("y"), y=w2157) -> (x-y=w2164:dbl)
        n1946 = expression code="10**y"(w2170) -> (w2150:dbl)
        n1947 = expression code="10**y"(w2164) -> (w2163:dbl)
        n1948 = Multiply(x=w2148, y=w2150) -> (x*y=w2149:dbl)
        n1949 = Multiply(x=w2161, y=w2163) -> (x*y=w2162:dbl)
        n1950 = Divide(x=w2149, y=750.0) -> (x/y=w2165:dbl)
        n1951 = Divide(x=w2162, y=750.0) -> (x/y=w2166:dbl)
        n1952 = Add(x=w2165, y=w2166) -> (x+y=w2167:dbl)
        n1953 = Divide(x=w2167, y=2.0) -> (x/y=w2169:dbl)
        n1954 = local write "AVP"(w2169) -> ()
        n1955 = Subtract(x=1.4, y=w2169) -> (x-y=w2152:dbl)
        n1956 = local read "HCF"() -> (w2153:dbl)
      }
      frame Enabled {
      }
    }
    n1957 = case shown="True" "EDIT 3" {
      frame False {
      }
      frame True {
        n1958 = local write "EDIT 3"(FALSE ("EDIT 3")) -> ()
        n1959 = local write "Main Tab"(T2."About" ("Main Tab")) -> ()
      }
    }
    n1960 = case shown="True" w2124 {
      frame False {
      }
      frame True {
        n1961 = local write "Re-Initialise"(FALSE ("Re-Initialise")) -> ()
      }
    }
    n1962 = case shown="False" w2138 {
      frame False {
        n1963 = local read "stopT"() -> (w3143:bool)
        n1964 = case shown="True" w3143 {
          frame False {
          }
          frame True {
            w3144 = FALSE
            n1965 = local write "stopT"(w3144) -> ()
            n1966 = local write "st enable"(w3144) -> ()
          }
        }
      }
      frame True {
        "stopT" <- TRUE
      }
    }
    n1967 = case shown="True" w2136 {
      frame False {
      }
      frame True {
      }
    }
    n1968 = case shown="True" w2126 {
      frame False {
        n1969 = property on="Password 2" class="Str"("Visible"=FALSE) -> ()  [unwired: 2 in, 2 out]
        n1970 = local write "Password 2"("" ("Password")) -> ()
      }
      frame True {
        n1971 = property on="Password 2" class="Str"("Visible"=TRUE) -> ()  [unwired: 2 in, 2 out]
        n1972 = Equal?(x="Password 2", y="HFRR1234") -> (x = y?=w2259:bool)
        n1973 = case shown="True" w2259 {
          tunnel: "Password 2" -> [w2262 _]
          frame False {
            n1974 = String Length(string=w2262) -> (length=w2263:i32)
            n1975 = Greater Than 0?(x=w2263) -> (x > 0?=w2261:bool)
            n1976 = case shown="False" w2261 {
              frame False {
                n1977 = property on="Password 2" class="Str"("Caption.Text"="Password (Advance Setting)") -> ()  [unwired: 2 in, 2 out]
              }
              frame True {
                n1978 = property on="Password 2" class="Str"("Caption.Text"="Incorrect Password!") -> ()  [unwired: 2 in, 2 out]
              }
            }
          }
          frame True {
            n1979 = local write "EDIT 2"(FALSE ("EDIT 2")) -> ()
            n1980 = local write "Password 2"("" ("Password")) -> ()
            n1981 = local write "Main Tab"(T2."Advance" ("Main Tab")) -> ()
            n1982 = local write "Main Dashboard Buttons"(T1."Advance" ("Main Dashboard Buttons")) -> ()
          }
        }
      }
    }
    n1983 = case shown="True" "Prog Uno" {
      frame False {
      }
      frame True {
        n1984 = stacked-sequence {
          frame #0 {
            n1985 = Delete(path (use dialog)=path "C:/LAB-IQ-NXT/UNOCOMPILE.bat" ("working directory")) -> ()  [unwired: 4 in, 3 out]
          }
          frame #1 {
            n1986 = local read "Com Port 1"() -> (w2724:refnum<visa-resource-name>)
            n1987 = Concatenate Strings("cmd.exe /c \"mode " ("command line"), w2724, ":1200,n,8,1\"\n" ("command line")) -> (w2729:string)
            n1988 = Concatenate Strings(w2729, "CD\\\nCD WinDucom\navrdude -C avrdude.conf -v -patmega328p -carduino -P" ("command line"), w2724, " -b115200 -D -Uflash:w:UNO_V20.hex:i\n" ("command line"), "\r") -> (w2731:string)
            "STR" <- w2731
            n1989 = call <vilib>:"Write Characters To File.vi"("append to file? (new file:F)"=FALSE, "character string"=w2731, "file path (dialog if empty)"=path "C:/LAB-IQ/UNOCOMPILE.bat" ("working directory")) -> ()  [unwired: 2 in, 1 out]
          }
          frame #2 {
            n1990 = disable-structure shown="Disabled" {
              frame Disabled {
                w2735 = "cmd.exe  /c \"C:\\LAB-IQ-NXT\\UNOCOMPILE.bat\"" ("string")
                n1991 = local write "Prog Uno"(FALSE ("run minimized? (F)")) -> ()
                n1992 = call <vilib>:"System Exec.vi"("expected output size  (4096)"=u32 65535, "run minimized? (F)"=FALSE, "wait until completion? (T)"=TRUE ("run minimized? (F)"), "working directory"=path "C:/LAB-IQ-NXT", "standard input"=w2735, "command line"=w2735) -> ("error out"=w2734:errorcluster, "standard output"=→"String 42":string)  [unwired: 2 in, 2 out]
                "error out 3" <- w2734
                n1993 = flat-sequence {
                  tunnel: w2734 -> [_]
                  frame #0 {
                  }
                }
              }
              frame Enabled {
              }
            }
          }
        }
      }
    }
    n1994 = case shown="\"CEC F-096-A-06\"" "TEST STANDARD" {
      tunnel: [2.0 ("Set Temp") 0.0 ("Set Temp") 2.0 ("Set Temp") 0.0 ("Set Temp")] -> w2127
      frame "ASTM D6079", Default {
        w2681 = 50.0 ("Hz")
        w2682 = 53.0 ("Set Rh")
        w2684 = 1.0 ("Set Strk")
        w2683 = 60.0 ("Set Temp")
        # "astm hide"
        n1995 = local write "NORMAL LOAD"(200.0 ("NORMAL LOAD")) -> ()
        n1996 = local write "Set Strk"(w2684) -> ()
        n1997 = local write "Set Hz"(w2681) -> ()
        n1998 = local write "Set Temp"(w2683) -> ()
        n1999 = local write "Set Rh"(w2682) -> ()
        n2000 = local write "test time"(75.0 ("test time")) -> ()
        n2001 = local write "Set Stroke:"(w2684) -> ()
        n2002 = local write "Set Humidity:"(w2682) -> ()
        n2003 = local write "Set Frequency:"(w2681) -> ()
        n2004 = local write "Set Temperature:"(w2683) -> ()
        "Test Standard" <- "ASTM D6079" ("Test Standard 2")
      }
      frame "ISO 12156" {
        n2005 = local write "Set Strk"(1.0 ("Set Strk")) -> ()
        n2006 = local write "NORMAL LOAD"(200.0 ("NORMAL LOAD")) -> ()
        n2007 = local write "Set Temp"(60.0 ("Set Temp")) -> ()
        n2008 = local write "test time"(75.0 ("test time")) -> ()
        n2009 = local write "Set Hz"(50.0 ("Hz")) -> ()
        n2010 = local write "Set Rh"(53.0 ("Set Rh")) -> ()
      }
      frame "CEC F-096-A-06" {
        n2011 = local write "Set Strk"(1.0 ("Set Strk")) -> ()
        n2012 = local write "NORMAL LOAD"(200.0 ("NORMAL LOAD")) -> ()
        n2013 = local write "Set Temp"(60.0 ("Set Temp")) -> ()
        n2014 = local write "test time"(75.0 ("test time")) -> ()
        n2015 = local write "Set Hz"(50.0 ("Hz")) -> ()
        n2016 = local write "Set Rh"(53.0 ("Set Rh")) -> ()
      }
      frame "Custom" {
      }
    }
    n2017 = case shown="True" "Prog Due" {
      frame False {
      }
      frame True {
        n2018 = stacked-sequence {
          frame #0 {
            n2019 = Delete(path (use dialog)=path "C:/LAB-IQ/DUECOMPILE.bat" ("working directory")) -> ()  [unwired: 4 in, 3 out]
          }
          frame #1 {
            n2020 = disable-structure shown="Disabled" {
              frame Disabled {
                n2021 = local read "visa due"() -> (w2706:string)
                n2022 = Concatenate Strings("cmd.exe /c \"mode " ("command line"), w2706, ":1200,n,8,1\"\n" ("command line")) -> (w2711:string)
                n2023 = Concatenate Strings(w2711, "CD\\\nCD WinDucom\nTIMEOUT 1\n bossac.exe -i -d --port=" ("command line"), w2706, " -U false -e -w -v -b DUE.bin -R\n" ("command line"), "\r") -> (w2713:string)
                "concatenated string 2" <- w2713
                n2024 = call <vilib>:"Write Characters To File.vi"("append to file? (new file:F)"=FALSE, "character string"=w2713, "file path (dialog if empty)"=path "C:/LAB-IQ-NXT/DUECOMPILE.bat" ("working directory")) -> ()  [unwired: 2 in, 1 out]
              }
              frame Enabled {
              }
            }
          }
          frame #2 {
            # "C:\\LAB-IQ-NXT\\DUECOMPILE.bat"
            n2025 = disable-structure shown="Disabled" {
              frame Disabled {
                w2718 = "cmd.exe  /c \"C:\\LAB-IQ-NXT\\DUECOMPILE.bat\"" ("string")
                n2026 = call <vilib>:"System Exec.vi"("expected output size  (4096)"=u32 65535, "run minimized? (F)"=FALSE, "wait until completion? (T)"=TRUE ("run minimized? (F)"), "working directory"=path "C:/LAB-IQ-NXT", "standard input"=w2718, "command line"=w2718) -> ("error out"=w2717:errorcluster, "standard output"=→"String 44":string)  [unwired: 2 in, 2 out]
                "error out 4" <- w2717
                n2027 = flat-sequence {
                  tunnel: w2717 -> [_]
                  frame #0 {
                  }
                }
              }
              frame Enabled {
              }
            }
            n2028 = local write "Prog Due"(FALSE ("Prog Due")) -> ()
          }
        }
      }
    }
    n2029 = Or(x=w2123, y=w2121) -> (x .or. y?=w2122:bool)
    n2030 = case shown="\"About\"" w2120 {
      tunnel: [T23."Acquire" ("Main Tab") T23."Compare Files" ("Main Tab") T23."About" ("Main Tab")] -> w2134
      frame "Acquire", Default {
      }
      frame "Compare Files" {
      }
      frame "About" {
      }
    }
    n2031 = Or(x=w2128, y="OPEN") -> (x .or. y?=w2129:bool)
    n2032 = case shown="True" w2129 {
      tunnel: w2128 -> [_ w2270]
      frame False {
      }
      frame True {
        n2033 = stacked-sequence {
          tunnel: w2270 -> [_ w2337 _ _]
          frame #0 {
            w2286 = "  " ("String 6")
            n2034 = local write "OPEN"(FALSE ("open")) -> ()
            n2035 = local read "string1 2"() -> (w2274:string)
            n2036 = local read "string1 3"() -> (w2273:string)
            n2037 = local read "string1 4"() -> (w2272:string)
            n2038 = property on="OPEN" class="Bool (strict)"("Visible"=FALSE) -> ()  [unwired: 2 in, 2 out]
            n2039 = local write "String 6"(w2286) -> ()
            n2040 = local write "String 7"(w2286) -> ()
            n2041 = local write "String 8"(w2286) -> ()
            n2042 = local write "String 12"(w2286) -> ()
            n2043 = local read "OK Button 16"() -> (w2271:bool)
            n2044 = String To Path(string=w2274) -> (path=w2282:path)
            n2045 = String To Path(string=w2273) -> (path=w2281:path)
            n2046 = String To Path(string=w2272) -> (path=w2280:path)
            n2047 = case shown="True" w2271 {
              tunnel: [w2287 w2288] -> w2275
              frame False {
                n2048 = local read "string1"() -> (w2287:string)
              }
              frame True {
                n2049 = local read "String Indicator 4"() -> (w2288:string)
              }
            }
            n2050 = Open/Create/Replace File "Open File"(file path (use dialog)=w2282) -> (refnum out=w2278:refnum<file>)  [unwired: 5 in, 2 out]
            n2051 = Open/Create/Replace File "Open File"(file path (use dialog)=w2281) -> (refnum out=w2277:refnum<file>)  [unwired: 5 in, 2 out]
            n2052 = Open/Create/Replace File "Open File"(file path (use dialog)=w2280) -> (refnum out=w2276:refnum<file>)  [unwired: 5 in, 2 out]
            n2053 = while {
              tunnel: w2278 -> [w2300]
              i -> [w2296]
              stop <- w2295 continue-if-true
              (unwired) TRUE ("line mode (F)")
              n2054 = Read from Text File "Read File"(file (use dialog)=w2300) -> (text=w2297:string)  [unwired: 3 in, 3 out]
              n2055 = local write "Numeric 11"(w2296) -> ()
              n2056 = String Length(string=w2297) -> (length=w2299:i32)
              n2057 = Greater?(x=w2299, y=1) -> (0:w2295:bool)
            }
            n2058 = while {
              tunnel: w2277 -> [w2306]
              i -> [w2302]
              stop <- w2301 continue-if-true
              (unwired) TRUE ("line mode (F)")
              n2059 = Read from Text File "Read File"(file (use dialog)=w2306) -> (text=w2303:string)  [unwired: 3 in, 3 out]
              n2060 = local write "Numeric 12"(w2302) -> ()
              n2061 = String Length(string=w2303) -> (length=w2305:i32)
              n2062 = Greater?(x=w2305, y=1) -> (0:w2301:bool)
            }
            n2063 = while {
              tunnel: w2276 -> [w2312]
              i -> [w2308]
              stop <- w2307 continue-if-true
              (unwired) TRUE ("line mode (F)")
              n2064 = Read from Text File "Read File"(file (use dialog)=w2312) -> (text=w2309:string)  [unwired: 3 in, 3 out]
              n2065 = local write "Numeric 13"(w2308) -> ()
              n2066 = String Length(string=w2309) -> (length=w2311:i32)
              n2067 = Greater?(x=w2311, y=1) -> (0:w2307:bool)
            }
            n2068 = String To Path(string=w2275) -> (path=w2283:path)
            n2069 = Open/Create/Replace File "Open File"(file path (use dialog)=w2283) -> (refnum out=w2279:refnum<file>)  [unwired: 5 in, 2 out]
            n2070 = while {
              tunnel: w2279 -> [w2294]
              i -> [w2290]
              stop <- w2289 continue-if-true
              (unwired) TRUE ("line mode (F)")
              n2071 = Read from Text File "Read File"(file (use dialog)=w2294) -> (text=w2291:string)  [unwired: 3 in, 3 out]
              n2072 = local write "Numeric 8"(w2290) -> ()
              n2073 = String Length(string=w2291) -> (length=w2293:i32)
              n2074 = Greater?(x=w2293, y=1) -> (0:w2289:bool)
            }
          }
          frame #1 {
            w2464 = FALSE ("ACTUAL   MERGE")
            # "Sample Temp"
            # "ECR"
            # "COF"
            # "Time\nCOF\nFF\nTemp"
            n2075 = case shown="True" w2337 {
              tunnel: [w2484 w2485] -> w2338
              frame False {
                n2076 = local read "string1"() -> (w2484:string)
              }
              frame True {
                n2077 = local read "String Indicator 4"() -> (w2485:string)
              }
            }
            n2078 = local read "string1 3"() -> (w2382:string)
            n2079 = String To Path(string=w2338) -> (path=w2469:path)
            n2080 = String To Path(string=w2382) -> (path=w2480:path)
            n2081 = local read "Numeric 12"() -> (w2466:i32)
            n2082 = local read "Numeric 8"() -> (w2468:i32)
            n2083 = local read "string1 2"() -> (w2383:string)
            n2084 = local read "string1 4"() -> (w2381:string)
            n2085 = Open/Create/Replace File "Open File"(file path (use dialog)=w2469) -> (refnum out=w2483:refnum<file>, error out=w2482:errorcluster)  [unwired: 5 in, 1 out]
            n2086 = Open/Create/Replace File "Open File"(file path (use dialog)=w2480) -> (refnum out=w2476:refnum<file>, error out=w2477:errorcluster)  [unwired: 5 in, 1 out]
            n2087 = for {
              N: w2468 -> [_]
              tunnel: w2483 -> [w2631]
              tunnel: w2482 -> [w2630]
              tunnel: [w2620] -> w2395 mode=indexing
              tunnel: [w2618] -> w2452 mode=indexing
              tunnel: [w2619] -> w2447 mode=indexing
              tunnel: w2464 -> [_]
              tunnel: [w2612] -> w2449 mode=indexing
              tunnel: [w2608] -> w2418 mode=indexing
              tunnel: [w2604] -> w2393 mode=indexing
              tunnel: [w2600] -> w2374 mode=indexing
              tunnel: [w2595] -> w2334 mode=indexing
              (unwired) TRUE ("line mode (F)")
              # "freq"
              # "Stroke"
              # "Time"
              # "CoF"
              # "Humidity"
              # "Temp"
              # "Air Temp"
              # "ECR"
              n2088 = Read from Text File "Read File"(file (use dialog)=w2631, error in=w2630) -> (text=w2596:string)  [unwired: 2 in, 3 out]
              n2089 = local write "String 6"(w2596) -> ()
              n2090 = String Subset(string=w2596, offset (0)=0, length (rest)=14 ("length (rest)")) -> (substring=w2624:string)
              n2091 = String Subset(string=w2596, offset (0)=35, length (rest)=9 ("length (rest)")) -> (substring=w2621:string)
              n2092 = String Subset(string=w2596, offset (0)=15, length (rest)=9 ("length (rest)")) -> (substring=w2627:string)
              n2093 = Fract/Exp String To Number(string=w2624) -> (number=w2620:dbl)  [unwired: 3 in, 1 out]
              n2094 = Fract/Exp String To Number(string=w2621) -> (number=w2619:dbl)  [unwired: 3 in, 1 out]
              n2095 = Fract/Exp String To Number(string=w2627) -> (number=w2618:dbl)  [unwired: 3 in, 1 out]
              n2096 = String Subset(string=w2596, offset (0)=85, length (rest)=9 ("length (rest)")) -> (substring=w2597:string)
              n2097 = String Subset(string=w2596, offset (0)=25, length (rest)=9 ("length (rest)")) -> (substring=w2603:string)
              n2098 = String Subset(string=w2596, offset (0)=55, length (rest)=9 ("length (rest)")) -> (substring=w2605:string)
              n2099 = String Subset(string=w2596, offset (0)=45, length (rest)=9 ("length (rest)")) -> (substring=w2611:string)
              n2100 = String Subset(string=w2596, offset (0)=65, length (rest)=9 ("length (rest)")) -> (substring=w2617:string)
              n2101 = Fract/Exp String To Number(string=w2603) -> (number=w2600:dbl)  [unwired: 3 in, 1 out]
              n2102 = Fract/Exp String To Number(string=w2597) -> (number=w2595:dbl)  [unwired: 3 in, 1 out]
              n2103 = Fract/Exp String To Number(string=w2605) -> (number=w2604:dbl)  [unwired: 3 in, 1 out]
              n2104 = Fract/Exp String To Number(string=w2611) -> (number=w2608:dbl)  [unwired: 3 in, 1 out]
              n2105 = Fract/Exp String To Number(string=w2617) -> (number=w2614:dbl)  [unwired: 3 in, 1 out]
              n2106 = Add(x=w2614, y=0.0) -> (x+y=w2612:dbl)
            }
            n2107 = for {
              N: w2466 -> [_]
              tunnel: w2477 -> [w2557]
              tunnel: w2476 -> [w2556]
              tunnel: [w2546] -> w2435 mode=indexing
              tunnel: [w2544] -> w2433 mode=indexing
              tunnel: [w2545] -> w2429 mode=indexing
              tunnel: w2464 -> [_]
              tunnel: [w2538] -> w2431 mode=indexing
              tunnel: [w2534] -> w2413 mode=indexing
              tunnel: [w2530] -> w2389 mode=indexing
              tunnel: [w2527] -> w2370 mode=indexing
              tunnel: [w2523] -> w2329 mode=indexing
              (unwired) 9 ("length (rest)")
              (unwired) 9 ("length (rest)")
              (unwired) TRUE ("line mode (F)")
              n2108 = Read from Text File "Read File"(file (use dialog)=w2556, error in=w2557) -> (text=w2524:string)  [unwired: 2 in, 3 out]
              n2109 = local write "String 8"(w2524) -> ()
              n2110 = String Subset(string=w2524, offset (0)=85) -> (substring=w2526:string)  [unwired: 1 in]
              n2111 = String Subset(string=w2524, offset (0)=35, length (rest)=9 ("length (rest)")) -> (substring=w2547:string)
              n2112 = String Subset(string=w2524, offset (0)=55, length (rest)=9 ("length (rest)")) -> (substring=w2532:string)
              n2113 = String Subset(string=w2524, offset (0)=25) -> (substring=w2528:string)  [unwired: 1 in]
